vi "Set Server Internal UEs.vi"(10 "Server Internal UEs":T1, 11 "OOP Server in":refnum<class "server12.lvclass">) -> (3 "OOP Server out":refnum<class "server12.lvclass">)   [LabVIEW 2020, in "server12.lvlib" / "server12.lvclass"]
uses:
  server12.lvclass
  typeDefs/Server Internal UEs.ctl
  server12.lvclass/server12.ctl
  typeDefs/Server Internal Message.ctl
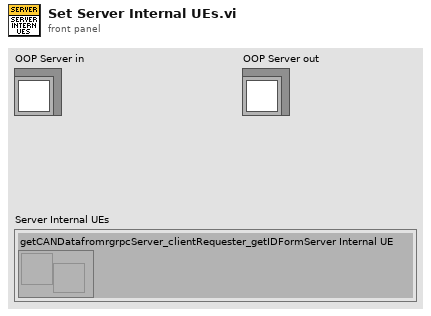
[diagram p1: front panel]
types:
  T1 = typedef "server12.lvlib/server12.lvclass/Server Internal UEs.ctl" = cluster{"getCANDatafromrgrpcServer_clientRequester_getIDFormServer Internal UE":refnum<user-event>}
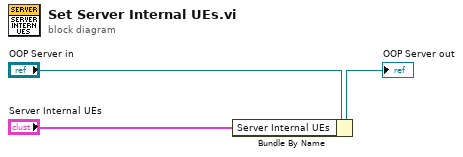
[diagram p0: block diagram]
diagram:
  n1 = Bundle By Name(cluster="OOP Server in", "Server Internal UEs"="Server Internal UEs") -> (→"OOP Server out":refnum<class "server12.lvclass">)
